vi "EnFlo_Tunnel_Setup.vi"() -> ()   [LabVIEW 2012]
uses:
  ADAM Controls/Ch_description_ADAM.ctl
  ADAM Controls/Module_type_ADAM.ctl
  ADAM Controls/Function_ADAM.ctl
  ADAM Controls/Channel_State.ctl
  ADAM Controls/Calib_type_ADAM.ctl
  ADAM Controls/Address.ctl
  ADAM Controls/Update_scan_value.ctl
panel:
  in  "Desired Lab Air Temp":dbl format="%.2f"
  out "Numerical Values":dbl[](array[numeric]) format="%.9f"
  out "Ch Description Array":T1[](array[typedef]) {"Duty" format="%.0b"; "D" format="%#_5g"; "C" format="%#_5g"; "B" format="%#_5g"; "A" format="%#_5g"}
  in  "Traverse Origin X Offset (mm)":dbl min=0.0 max=20000.0
  in  "Show Heater Setup":bool
  in  "stop":bool
  in  "Desired Chilled Water Temp":dbl format="%.2f"
  out "Reference Anemometer":string
  in  "OK":bool
  in  "Obstacle Orientation (Deg)":dbl format="%.2f"
  in  "Obstacle/Building":u16(ring) items=["1-500 DAPPLE low Res", "100mm Trench", "100x100 Cube", "100x100 pressure tapped cube", "100x100x200 Tall", "100x100x300 Tall", "100x100x400mm Tall", "110mm cube array 110mm spacing", "110mm cube array 55mm spacing", "12 WTs", "150*150*150mm cube", "16 blocks 55 x 55 x 110mm tall centre at x=12m", "16 buildings 250*500*125mm", "16 x 110mm cube array 110mm spacing", "20 buildings 500x250x125mm", "25 x 110mm cube array 110mm spacing", "25mm Trench in 1.4m Turntable", "4 buildings 750x500x125mm", "4 x 110mm cube array 110mm spacing", "400mm x 400mm Heated Mat centre 12m", "500x250x125 Block", "660mm x 3000mm Heated Mat centre 12m", "9 x 110mm cube array 110mm spacing", "990mm x 3000mm Heated Mat centre 14m", "Array of 24 tanks dia 130mm height 88mm", "Blade 1", "Blade 2", "Building With Single Stack", "Building with Twin Stack", "Concawe Actual Model 6 Cylinders", "DAPPLE high Res buildings at intersection", "DAPPLE low Res", "DAPPLE low Res with roof roughness", "DAPPLE low Res(model+B42-45 and obstacles in the west of the model)", "DAPPLE low Res(sampling at Mary  Rd  Model+B42-45)", "DAPPLE low Res(sampling at Mary  Rd with B38-41and A5)", "DAPPLE low Res(sampling at Mary  Rd without B38-41)", "DAPPLE low Res(sampling at Mary. Rd add A1-5)", "DYCE_London_110mm", "False Floor (table 4.17m x 0.9m  height 230mm)", "Forest at x=11003", "Group of 2 Tanks D=133mm upstream tank", "Group of 6 Tanks D=400mm no downstream tanks", "Group of 9 Tanks D=133mm Centre releasing 67mm roof heights", "Group of 9 Tanks D=400mm 3 downstream tanks", "HRModUrb SimpleC", "HRModUrb SimpleC with tall building", "HRModUrb SimpleV", "Headstart07 building", "Network Regular", "None", "Norway 1:300", "Norway 1:500", "ROSE (Bremen)", "Row_of_blocks_H=204_L=250mm", "Sellafiield Site Model", "Sellafiield Site Model (Flat)", "Single Turbine II", "Single wind turbine (blade II) at X=10000 Y=0", "St Thomas Hospital - East Wing - Unclad", "St Thomas Hospital - East Wing - clad", "Storage Tank H=100  D=400mm", "Storage Tank H=100  D=400mm with 0 Deg Bund", "Storage Tank H=100  D=400mm with 45 Deg Bund", "Storage Tank H=100  D=400mm with Bund plus upstream tank", "Storage Tank H=100 D=500mmStorage Tank H=100  D=700mm", "Storage Tank H=89  D=133mm", "Storage Tank H=89  D=133mm with 0 Deg Bund", "Storage Tank H=89  D=133mm with 266mm Bund on turn table", "Storage Tank H=89  D=133mm with 45 Deg Bund", "Subfloor trench 285x285x3m", "Tree 171 mm - Dense", "Tree 171 mm - Porous", "Tree 91 mm - Dense", "Tree 91 mm - Porous", "Tree85mmRow - x=13000", "Vehicle 1to20 - False Floor (table 4.17m x 0.9m  height 230mm)", "Vehicle 1to5 - False Floor (table 4.17m x 0.9m  height 230mm)", "WT Array1", "WT Array2", "WT Array21", "WT Array3", "WT Array4", "WT Array5", "WT Array6", "WT Array7", "WT x 2", "WT x 3", "WT x 4", "Edit Strings"]
  in  "Vorticity Generators":u16(ring) items=["5 Irwin spires 1.2m   X=50mm", "Not Installed", "Offshore 5x TruncIrwin (H:1490)  B(H:0):150  B(H:1490):10  Yspace:660  X:50", "Offshore 5x TruncIrwin (H:1490)  B(H:0):150  B(H:700):10  Yspace:660  X:50", "Offshore+onshore", "Onshore 5xTruncNonIrwin (H:1490  B(H:0-120):250  B(H:192):177  B(H:1490):24)  YSpace:660 X:50", "Edit Strings"]
  in  "Side Wall Separation":u16(ring) items=["1.07m", "1.5m", "2.0m", "2.5m", "2.93m", "3m  from x=0.67 to x=10.67m", "3m  from x=0.67 to x=12.67m", "3m  from x=0.67 to x=18m", "3m  from x=0.67 to x=6.67m", "3m  from x=8 to x=18m", "No sidewalls installed", "Edit Strings"]
  in  "Roughness Height":u16(ring) items=["H=16mm  W=50mm Yspace=510mm Xspace=360mm Staggered", "H=20mm W=80mm YSpace=240mm  XSpace=240mm Staggered", "H=20mm W=80mm YSpace=240mm  XSpace=720mm Staggered", "no roughness elements (smooth)", "Edit Strings"]
  in  "Job Name":u16(ring) items=["20 buildings 500x250x125mm", "ACTUAL", "Antonio_LDA_FFID_Neutral", "Building Wakes", "CONCAWE", "Convective_BL", "Cube", "DAPPLE", "DSTL", "DYCE", "Dense Gas", "Flow Uniformity", "Flying FFID Trials", "Gravity Waves", "HRModUrb", "Headstart07", "Home Office", "L Shaped Building", "LDA_tall_building_wake", "Line Source release", "Nantes Canyon", "Norway", "Odour", "ROSE", "Reference Dispersion", "Sandia 08", "Sellafield Jan 03", "Sellafield March 02", "Shell", "Silsoe Cube", "St Thomas Hospital", "Stable_Boundary_Layer", "Storage tanks", "Street Canyon", "Street Junction", "Supergen", "Tall Bldgs Disp", "Twin Stack Dispersion", "Vehicle_Wake", "Westlakes_08", "Westlakes_SAV2 WD=94", "XW_LDA_Comparison", "Edit Strings"]
  # "Boundary Layer Generation setup"
  # "This value should be zero if working in tunnel coordinates  (X=0 at start of working section)"
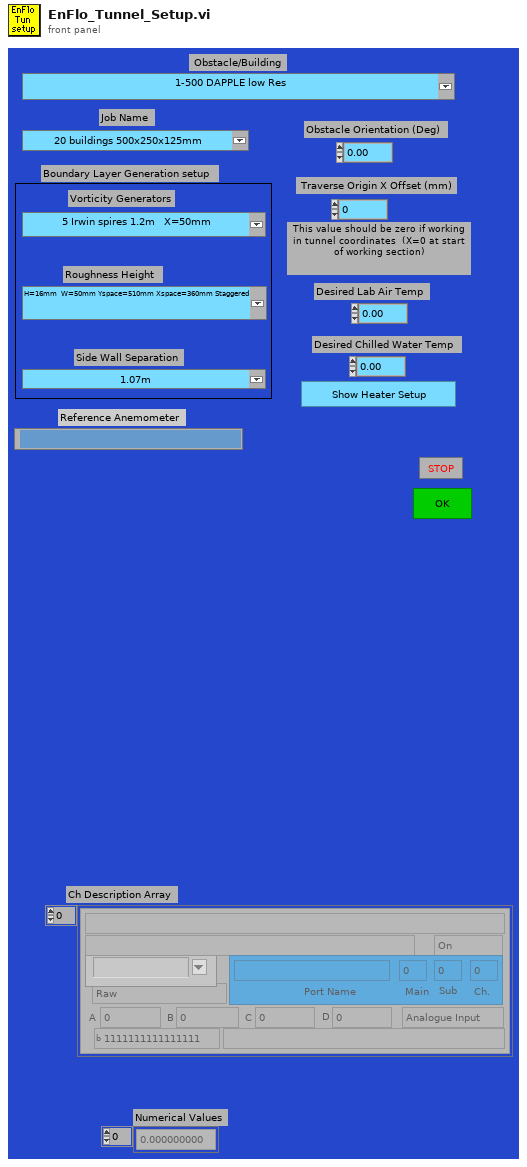
[diagram p1: front panel]
types:
  T1 = typedef "Ch_description_ADAM.ctl" = cluster{"Ch Name":string, "Type":T2, "Function":T3, "Ch State":T4, "Calibration type":T5, "A":dbl, "B":dbl, "C":dbl, "D":dbl, "Comments":string, "Address":T6, "String":string, "Duty":u16}
  T2 = typedef "Module_type_ADAM.ctl" = string
  T3 = typedef "Function_ADAM.ctl" = enum16{"Analogue Input", "Digital Input", "Event counter", "Event rate", "Analogue Output", "Digital Output", "Relay Output"}
  T4 = typedef "Channel_State.ctl" = enum16{"On", "Off", "Always On", "Always Off"}
  T5 = typedef "Calib_type_ADAM.ctl" = enum16{"Raw", "Bx + A", "Cx^2 + Bx + A", "Dx^3 + Cx^2 + Bx + A", "In Band", "Hi-Tec Q", "Hi-Tec M_dot", "Text"}
  T6 = typedef "Address.ctl" = cluster{"Main":i32, "Ch.":i32, "Sub":i32, "Port Name":string}
  T7 = typedef "Status_Cluster.ctl" = cluster{"Status":T8, "Error Type":string, "Error Description":string}
  T8 = typedef "Multi_Run_Status.ctl" = enum16{"Continue", "Jump to Next Point", "Jump to Next Row", "Jump To Fall Back", "Terminate Run"}
  T9 = typedef "Update_scan_value.ctl" = cluster{"Channel Name":string, "New Value":dbl}
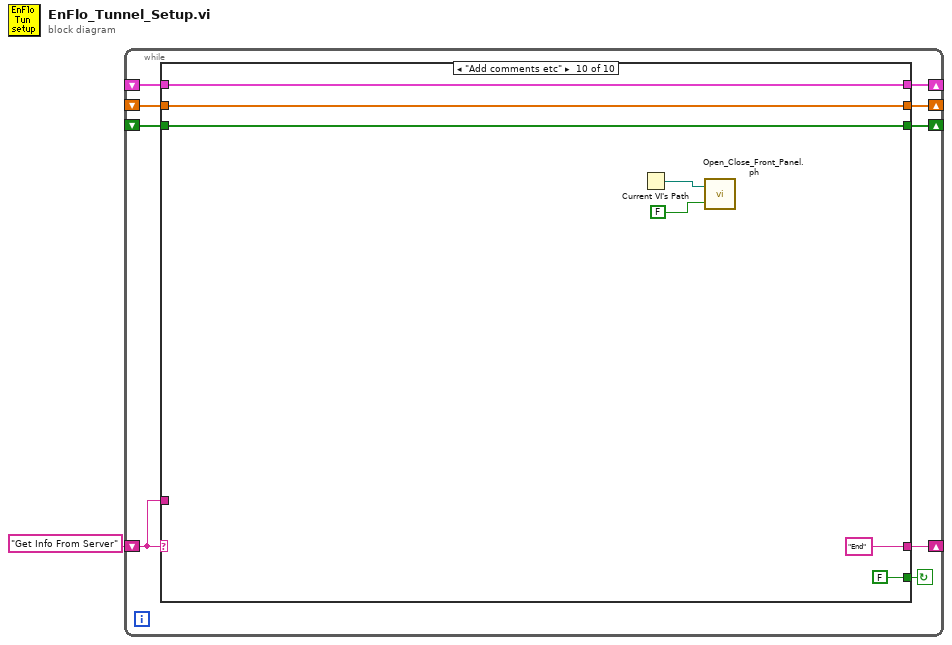
[diagram p0: block diagram]
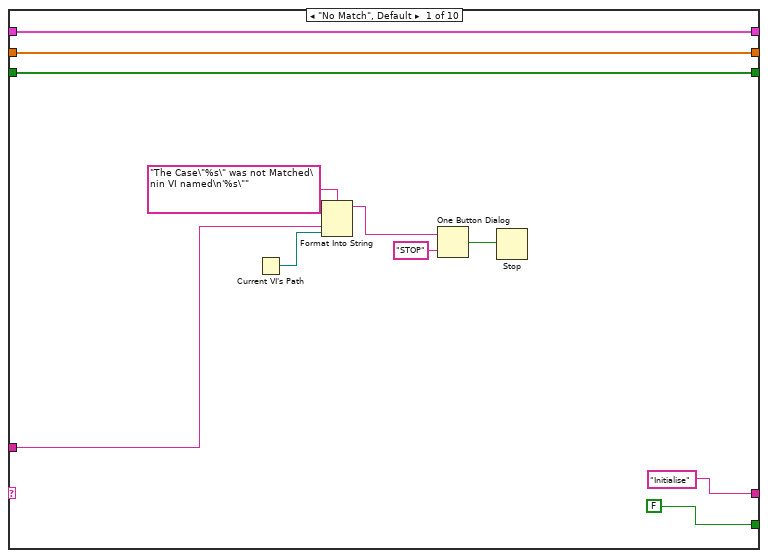
[diagram p2: hidden frame]
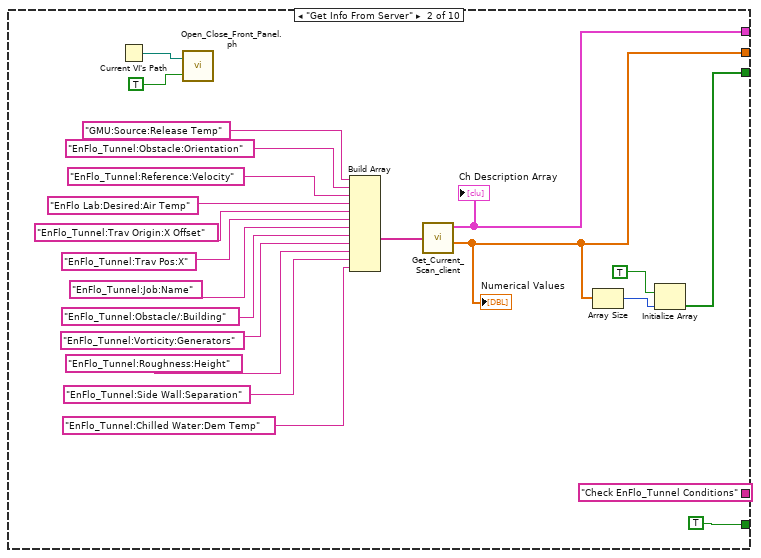
[diagram p3: hidden frame]
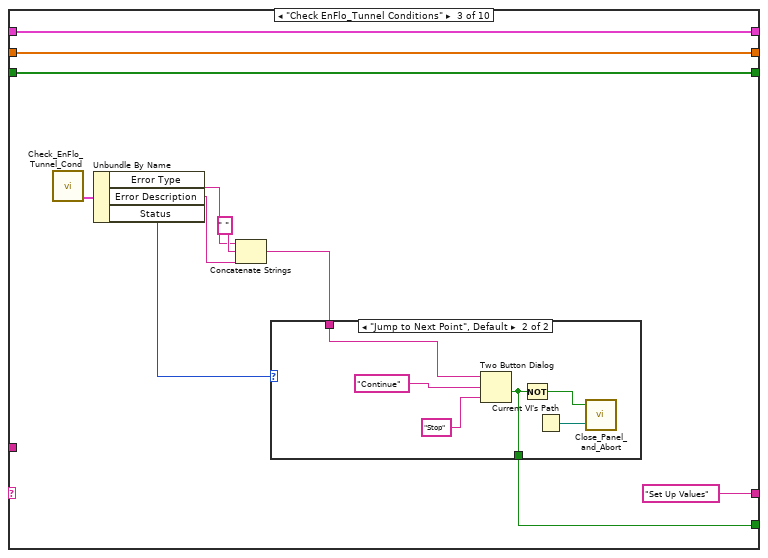
[diagram p4: hidden frame]
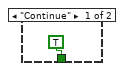
[diagram p5: hidden frame]
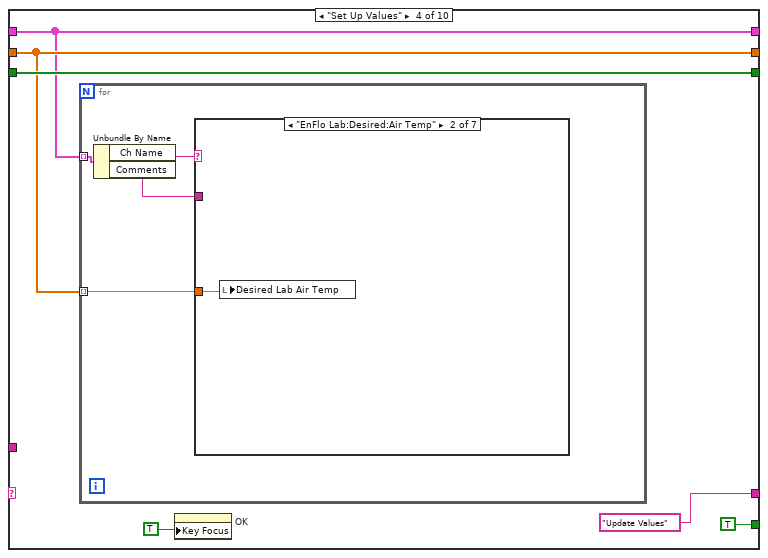
[diagram p6: hidden frame]
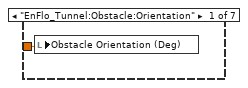
[diagram p7: hidden frame]
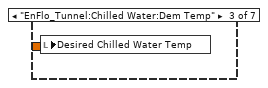
[diagram p8: hidden frame]
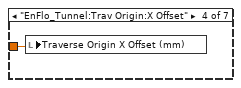
[diagram p9: hidden frame]
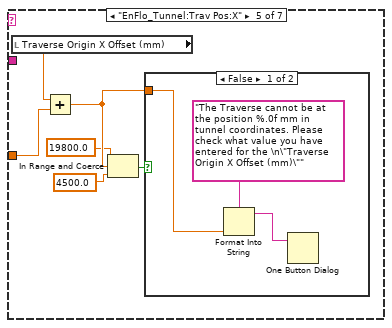
[diagram p10: hidden frame]
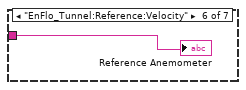
[diagram p12: hidden frame]
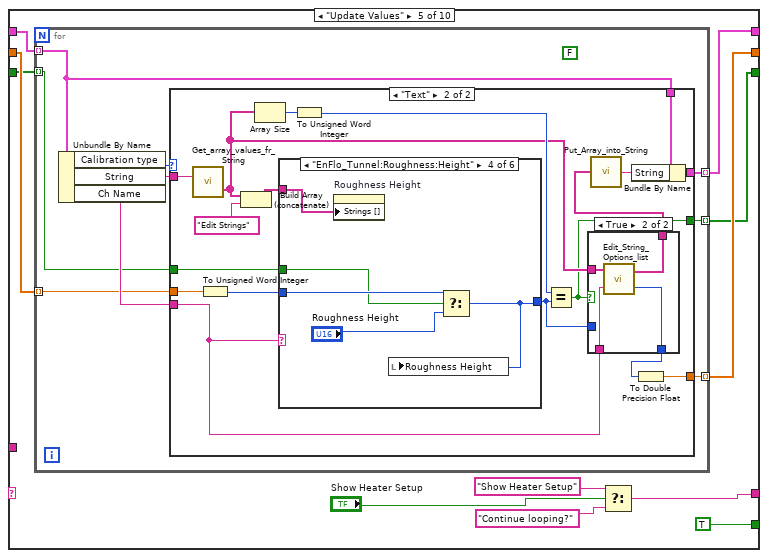
[diagram p14: hidden frame]
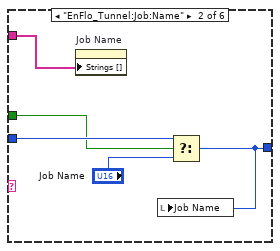
[diagram p18: hidden frame]
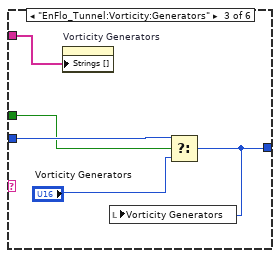
[diagram p19: hidden frame]
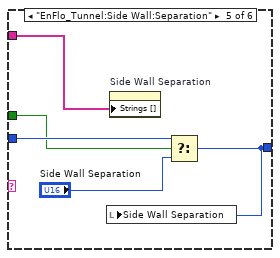
[diagram p20: hidden frame]
diagram:
  n1 = while {
    shift-left: _ -> [w2]
    shift-right: [w3] -> _
    shift-left: _ -> [w4]
    shift-right: [w6] -> _
    shift-left: _ -> [w5]
    shift-right: [w7] -> _
    shift-left: "Get Info From Server" -> [w8]
    shift-right: [w9] -> _
    stop <- w10 continue-if-true
    n2 = case shown="\"Add comments etc\"" w8 {
      tunnel: [FALSE TRUE w46 TRUE ("T button?") TRUE ("T button?") TRUE ("T button?") TRUE ("T button?") TRUE ("T button?") TRUE ("T button?") FALSE ("T button?")] -> w10
      tunnel: ["Initialise" "Check EnFlo_Tunnel Conditions" "Set Up Values" "Update Values" w90 "Continue looping?" w169 "Update Server" "Add comments etc" "End"] -> w9
      tunnel: w8 -> [w16 _ _ _ _ _ _ _ _ _]
      tunnel: [w13 w34 w48 w63 w94 w167 w178 w179 w211 w255] -> w7
      tunnel: [w12 w33 w47 w64 w92 w166 w177 w182 w210 w254] -> w6
      tunnel: w5 -> [w13 _ w48 w63 w95 w167 w178 w180 w211 w255]
      tunnel: w4 -> [w12 _ w47 w64 w93 w166 w177 w181 w210 w254]
      tunnel: [w11 w30 w44 w66 w86 w163 w175 w184 w209 w252] -> w3
      tunnel: w2 -> [w11 _ w44 w66 w87 w163 w175 w184 w209 w252]
      frame "No Match", Default {
        n3 = Current VI's Path() -> (path=w15:path)
        n4 = Format Into String(format string="The Case\"%s\" was not Matched\nin VI named\n'%s\"" ("Format String"), w16, w15) -> (resulting string=w19:string)  [unwired: 2 in, 1 out]
        n5 = One Button Dialog(message=w19, button name ("OK")="STOP") -> (true=w17:bool)
        n6 = Stop(stop? (T)=w17) -> ()
      }
      frame "Get Info From Server" {
        n7 = Current VI's Path() -> (path=w28:path)
        n8 = call "Open_Close_Front_Panel.ph.vi"("Front Panel Window:Open"=TRUE, "VI path"=w28) -> ()  [unwired: 2 out]
        n9 = Build Array("GMU:Source:Release Temp", "EnFlo_Tunnel:Obstacle:Orientation", "EnFlo_Tunnel:Reference:Velocity", "EnFlo Lab:Desired:Air Temp", "EnFlo_Tunnel:Trav Origin:X Offset", "EnFlo_Tunnel:Trav Pos:X", "EnFlo_Tunnel:Job:Name", "EnFlo_Tunnel:Obstacle/:Building", "EnFlo_Tunnel:Vorticity:Generators", "EnFlo_Tunnel:Roughness:Height", "EnFlo_Tunnel:Side Wall:Separation", "EnFlo_Tunnel:Chilled Water:Dem Temp") -> (w41:string[])
        n10 = call "Get_Current_Scan_client.vi"("ADAM Ch Names"=w41) -> ("Ch Description Array"=w34:T1[], "Numerical Values"=w33:dbl[])  [unwired: 2 out]
        "Ch Description Array" <- w34
        "Numerical Values" <- w33
        n11 = Array Size(array=w33) -> (size(s)=w32:i32)
        n12 = Initialize Array(TRUE, w32) -> (w30:bool[])
      }
      frame "Check EnFlo_Tunnel Conditions" {
        n13 = call "Check_EnFlo_Tunnel_Cond.vi"() -> ("Status Cluster"=w49:T7)  [unwired: 2 in, 1 out]
        n14 = Unbundle By Name(w49) -> ("Error Type"=w50:string, "Error Description"=w53:string, "Status"=w54:T8)
        n15 = Concatenate Strings(w50, " " ("Substring"), w53) -> (w52:string)
        n16 = case shown="\"Jump to Next Point\", Default" w54 {
          tunnel: w52 -> [_ w61]
          tunnel: [TRUE ("T button?") w57] -> w46
          frame "Continue" {
          }
          frame "Jump to Next Point", Default {
            n17 = Two Button Dialog(message=w61, 1:"Stop" ("F button name (\"Cancel\")"), 2:"Continue" ("T button name (\"OK\")")) -> (T button?=w57:bool)
            n18 = Not(x=w57) -> (.not. x?=w58:bool)
            n19 = Current VI's Path() -> (path=w59:path)
            n20 = call "Close_Panel_and_Abort.vi"("Vi path"=w59, "stop"=w58) -> ()  [unwired: 1 out]
          }
        }
      }
      frame "Set Up Values" {
        n21 = for {
          tunnel: w64 -> [w71] mode=indexing
          tunnel: w63 -> [w70] mode=indexing
          n22 = Unbundle By Name(w70) -> ("Ch Name"=w69:string, "Comments"=w68:string)
          n23 = case shown="\"EnFlo Lab:Desired:Air Temp\"" w69 {
            tunnel: w71 -> [w72 w73 w74 w75 w80 _ _]
            tunnel: w68 -> [_ _ _ _ _ w85 _]
            frame "EnFlo_Tunnel:Obstacle:Orientation" {
              n24 = local write "Obstacle Orientation (Deg)"(w72) -> ()
            }
            frame "EnFlo Lab:Desired:Air Temp" {
              n25 = local write "Desired Lab Air Temp"(w73) -> ()
            }
            frame "EnFlo_Tunnel:Chilled Water:Dem Temp" {
              n26 = local write "Desired Chilled Water Temp"(w74) -> ()
            }
            frame "EnFlo_Tunnel:Trav Origin:X Offset" {
              n27 = local write "Traverse Origin X Offset (mm)"(w75) -> ()
            }
            frame "EnFlo_Tunnel:Trav Pos:X" {
              n28 = local read "Traverse Origin X Offset (mm)"() -> (w81:dbl)
              n29 = Add(x=w81, y=w80) -> (x+y=w79:dbl)
              n30 = In Range and Coerce(upper limit=19800.0 ("y"), x=w79, lower limit=4500.0 ("y")) -> (In Range?=w76:bool)  [unwired: 1 out]
              n31 = case shown="False" w76 {
                tunnel: w79 -> [w84 _]
                frame False {
                  n32 = Format Into String(format string="The Traverse cannot be at the position %.0f mm in tunnel coordinates. Please check what value you have entered for the \n\"Traverse Origin X Offset (mm)\"" ("Format String"), w84) -> (resulting string=w82:string)  [unwired: 2 in, 1 out]
                  n33 = One Button Dialog(message=w82) -> ()  [unwired: 2 out]
                }
                frame True {
                }
              }
            }
            frame "EnFlo_Tunnel:Reference:Velocity" {
              "Reference Anemometer" <- w85
            }
            frame "No Match", Default {
            }
          }
        }
        n34 = property on="OK" class="Bool"("Key Focus"=TRUE ("Write Attribute")) -> ()  [unwired: 2 in, 2 out]
      }
      frame "Update Values" {
        n35 = for {
          tunnel: w95 -> [w102] mode=indexing
          tunnel: [w101] -> w94 mode=indexing
          tunnel: w93 -> [w100] mode=indexing
          tunnel: [w99] -> w92 mode=indexing
          tunnel: w87 -> [w98] mode=indexing
          tunnel: [w97] -> w86 mode=indexing
          (unwired) FALSE
          n36 = Unbundle By Name(w102) -> ("Calibration type"=w105:T5, "String"=w104:string, "Ch Name"=w103:string)
          n37 = case shown="\"Text\"" w105 {
            tunnel: w104 -> [_ w126]
            tunnel: w103 -> [_ w116]
            tunnel: w102 -> [w108 w120]
            tunnel: [w108 w119] -> w101
            tunnel: w100 -> [w107 w118]
            tunnel: [w107 w117] -> w99
            tunnel: w98 -> [w106 w115]
            tunnel: [w106 w109] -> w97
            frame "Raw", Default {
            }
            frame "Text" {
              n38 = call "Get_array_values_fr_String.vi"("String Value"=w126) -> ("String array"=w114:string[])  [unwired: 1 out]
              n39 = To Unsigned Word Integer(number=w118) -> (unsigned 16bit integer=w124:u16)
              n40 = Build Array (concatenate)(w114, "Edit Strings") -> (w113:string[])
              n41 = Array Size(array=w114) -> (size(s)=w125:i32)
              n42 = case shown="\"EnFlo_Tunnel:Roughness:Height\"" w116 {
                tunnel: [w133 w136 w141 w146 w150 w158] -> w110
                tunnel: w113 -> [_ w135 w140 w145 w151 w160]
                tunnel: w124 -> [w133 w137 w143 w148 w153 w161]
                tunnel: w115 -> [_ w134 w139 w144 w149 w154]
                frame "No match", Default {
                }
                frame "EnFlo_Tunnel:Job:Name" {
                  n43 = property on="Job Name" class="Ring (strict)"("Strings []"=w135) -> ()  [unwired: 2 in, 2 out]
                  n44 = Select(t=w137, s=w134, f="Job Name") -> (s? t:f=w136:u16)
                  n45 = local write "Job Name"(w136) -> ()
                }
                frame "EnFlo_Tunnel:Vorticity:Generators" {
                  n46 = property on="Vorticity Generators" class="Ring (strict)"("Strings []"=w140) -> ()  [unwired: 2 in, 2 out]
                  n47 = Select(t=w143, s=w139, f="Vorticity Generators") -> (s? t:f=w141:u16)
                  n48 = local write "Vorticity Generators"(w141) -> ()
                }
                frame "EnFlo_Tunnel:Roughness:Height" {
                  n49 = property on="Roughness Height" class="Ring (strict)"("Strings []"=w145) -> ()  [unwired: 2 in, 2 out]
                  n50 = Select(t=w148, s=w144, f="Roughness Height") -> (s? t:f=w146:u16)
                  n51 = local write "Roughness Height"(w146) -> ()
                }
                frame "EnFlo_Tunnel:Side Wall:Separation" {
                  n52 = property on="Side Wall Separation" class="Ring (strict)"("Strings []"=w151) -> ()  [unwired: 2 in, 2 out]
                  n53 = Select(t=w153, s=w149, f="Side Wall Separation") -> (s? t:f=w150:u16)
                  n54 = local write "Side Wall Separation"(w150) -> ()
                }
                frame "EnFlo_Tunnel:Obstacle/:Building" {
                  n55 = property on="Obstacle/Building" class="Ring (strict)"("Strings []"=w160) -> ()  [unwired: 2 in, 2 out]
                  n56 = Select(t=w161, s=w154, f="Obstacle/Building") -> (s? t:f=w158:u16)
                  n57 = local write "Obstacle/Building"(w158) -> ()
                  n58 = Index Array(array=w160, index=w158) -> (element=w155:string)
                  n59 = Not Equal?(x="None", y=w155) -> (x != y?=w156:bool)
                  n60 = property on="Obstacle Orientation" class="DigNum (strict)"("Visible"=w156) -> ()  [unwired: 2 in, 2 out]
                }
              }
              n61 = To Unsigned Word Integer(number=w125) -> (unsigned 16bit integer=w123:u16)
              n62 = Equal?(x=w123, y=w110) -> (x = y?=w109:bool)
              n63 = case shown="True" w109 {
                tunnel: w114 -> [w128 w132]
                tunnel: w116 -> [_ w131]
                tunnel: [w128 w130] -> w121
                tunnel: [w127 w129] -> w111
                tunnel: w110 -> [w127 _]
                frame False {
                }
                frame True {
                  n64 = call "Edit_String_Options_list.vi"("Channel Name"=w131, "String array"=w132) -> ("New Selection Index"=w129:i32, "String array Out"=w130:string[])
                }
              }
              n65 = call "Put_Array_into_String.vi"("String array"=w121) -> ("String Value"=w122:string)
              n66 = Bundle By Name(cluster=w120, "String"=w122) -> (w119:T1)
              n67 = To Double Precision Float(number=w111) -> (double precision float=w117:dbl)
            }
          }
        }
        n68 = Select(t="Show Heater Setup", s="Show Heater Setup", f="Continue looping?") -> (s? t:f=w90:string)
      }
      frame "Show Heater Setup" {
        n69 = call "Heater_Setpoint_Panel.vi"() -> ()  [unwired: 1 out]
        n70 = local write "Show Heater Setup"(FALSE ("Show Inlet heater Setup")) -> ()
      }
      frame "Continue looping?" {
        n71 = Or(x="stop", y="OK") -> (x .or. y?=w172:bool)
        n72 = Current VI's Path() -> (path=w174:path)
        n73 = call "Close_Panel_and_Abort.vi"("Vi path"=w174, "stop"="stop") -> ()  [unwired: 1 out]
        n74 = Select(t="Insert Values", s=w172, f="Update Values") -> (s? t:f=w169:string)
      }
      frame "Insert Values" {
        n75 = for {
          tunnel: w180 -> [w187] mode=indexing
          tunnel: w181 -> [w189] mode=indexing
          tunnel: [w188] -> w182 mode=indexing
          tunnel: [w186] -> w179 mode=indexing
          n76 = Unbundle By Name(w187) -> ("Ch Name"=w190:string)
          n77 = case shown="\"EnFlo_Tunnel:Chilled Water:Dem Temp\"" w190 {
            tunnel: w189 -> [_ _ _ _ w203]
            tunnel: ["Desired Lab Air Temp" "Desired Chilled Water Temp" "Traverse Origin X Offset (mm)" w198 w203] -> w188
            tunnel: w187 -> [w192 w194 w195 w197 w202]
            tunnel: [w192 w194 w195 w197 w202] -> w186
            frame "EnFlo Lab:Desired:Air Temp" {
            }
            frame "EnFlo_Tunnel:Chilled Water:Dem Temp" {
            }
            frame "EnFlo_Tunnel:Trav Origin:X Offset" {
            }
            frame "EnFlo_Tunnel:Obstacle:Orientation" {
              n78 = property on="Obstacle Orientation" class="DigNum (strict)"() -> ("Visible"=w201:bool)  [unwired: 2 in, 2 out]
              n79 = Not(x=w201) -> (.not. x?=w200:bool)
              n80 = call "Hide_Channel_value.vi"("Hide Values"=w200, "Value In"="Obstacle Orientation (Deg)") -> ("Value Out"=w198:dbl)  [unwired: 1 in]
            }
            frame "No Match", Default {
            }
          }
        }
      }
      frame "Update Server" {
        w206 = T9 {"Channel Name"="", "New Value"=0.0} ("Update Scan Value Cluster")
        n81 = Index Array(array=w211, index=0 ("Index")) -> (element=w222:T1)
        n82 = local read "Ch Description Array"() -> (w208:T1[])
        n83 = local read "Numerical Values"() -> (w207:dbl[])
        n84 = Initialize Array(w222, 0 ("Dimension Size")) -> (w220:T1[])
        n85 = Initialize Array(w206, 0 ("Dimension Size")) -> (w215:T9[])
        n86 = for {
          shift-right: [w235] -> w217
          shift-left: w220 -> [w236]
          tunnel: w211 -> [w226] mode=indexing
          shift-right: [w234] -> w212
          shift-left: w215 -> [w233]
          tunnel: w210 -> [w228] mode=indexing
          tunnel: w208 -> [w227] mode=indexing
          tunnel: w207 -> [w231] mode=indexing
          tunnel: w206 -> [w229]
          n87 = Equal?(x=w226, y=w227) -> (x = y?=w232:bool)
          n88 = Equal?(x=w228, y=w231) -> (x = y?=w230:bool)
          n89 = case shown="False" w230 {
            tunnel: w233 -> [w243 w244]
            tunnel: [w242 w244] -> w234
            tunnel: w229 -> [w241 _]
            tunnel: w228 -> [w240 _]
            tunnel: w226 -> [w239 _]
            frame False {
              n90 = Unbundle By Name(w239) -> ("Ch Name"=w238:string)
              n91 = Bundle By Name(cluster=w241, "Channel Name"=w238, "New Value"=w240) -> (w237:T9)
              n92 = Build Array (concatenate)(w243, w237) -> (w242:T9[])
            }
            frame True {
            }
          }
          n93 = case shown="False" w232 {
            tunnel: w236 -> [w247 w248]
            tunnel: w226 -> [w246 _]
            tunnel: [w245 w248] -> w235
            frame False {
              n94 = Build Array (concatenate)(w247, w246) -> (w245:T1[])
            }
            frame True {
            }
          }
        }
        n95 = Array Size(array=w217) -> (size(s)=w219:i32)
        n96 = Array Size(array=w212) -> (size(s)=w213:i32)
        n97 = Greater Than 0?(x=w219) -> (x > 0?=w218:bool)
        n98 = Greater Than 0?(x=w213) -> (x > 0?=w214:bool)
        n99 = case shown="True" w218 {
          tunnel: w217 -> [_ w225]
          frame False {
          }
          frame True {
            n100 = call "Update_Ch_Discription_client.vi"("Channels to update In"=w225) -> ()  [unwired: 1 out]
          }
        }
        n101 = case shown="True" w214 {
          tunnel: w212 -> [_ w224]
          frame False {
          }
          frame True {
            n102 = call "Update_Current_Value_client.vi"("Update array in"=w224) -> ()  [unwired: 1 in]
          }
        }
      }
      frame "Add comments etc" {
        n103 = Current VI's Path() -> (path=w249:path)
        n104 = call "Open_Close_Front_Panel.ph.vi"("Front Panel Window:Open"=FALSE, "VI path"=w249) -> ()  [unwired: 2 out]
      }
    }
  }
